vi "OnFontOrLocaleChange.vi"(0 "XRef":T10, 1 "State In":T1 {"BlockNodeState"."Draw Style" items=["FunctionBlock", "ExpressVI", "Variable", "Elemental I/O", "32x32 Icon", "FunctionBlockCompact"]; "BlockNodeState"."Terminal Data"."Terminal Flags" format="%.0b"}) -> (14 "Reply":T8, 15 "State Out":T1 {"BlockNodeState"."Draw Style" items=["FunctionBlock", "ExpressVI", "Variable", "Elemental I/O", "32x32 Icon", "FunctionBlockCompact"]; "BlockNodeState"."Terminal Data"."Terminal Flags" format="%.0b"})   [LabVIEW 2017, in "ExpressFormulaBlockNode.xnode"]
uses:
  <vilib>/express/express arith-compare/Formula/XNode/ExpressFormulaBlockNode.xnode
  <vilib>/XNodeSupport/XNodeXNodeRef.ctl
  <vilib>/express/express arith-compare/Formula/XNode/State.ctl
  <vilib>/BlockNodeSupport/BlockNodeState.ctl
  <vilib>/BlockNodeSupport/TerminalData.ctl
  <vilib>/picture/picture.llb/imagedata.ctl
  <vilib>/express/express shared/XNodes/controls/ExpressState.ctl
  <vilib>/express/express shared/XNodes/controls/ExpressTerminalInfo.ctl
  <vilib>/XNodeSupport/XNodeType.ctl
  <vilib>/XNodeSupport/XNodeStringArray.ctl
  <vilib>/XNodeSupport/XNodeString.ctl
  <vilib>/XNodeSupport/NI_XNodeSupport.lvlib
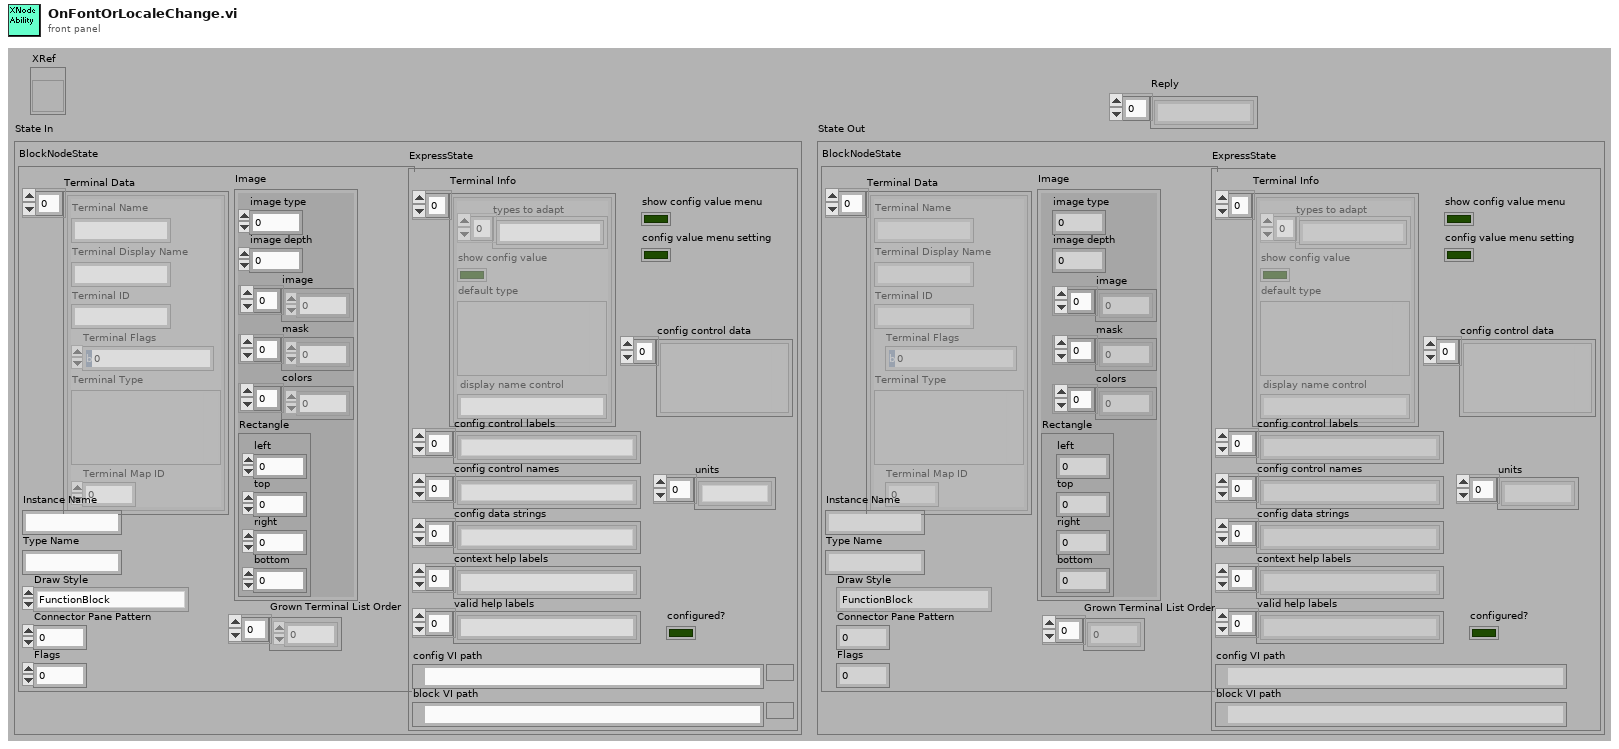
[diagram p1: front panel]
types:
  T1 = typedef "ExpressFormulaBlockNode.xnode/State.ctl" = cluster{"BlockNodeState":T2, "ExpressState":T5}
  T2 = typedef "BlockNodeState.ctl" = cluster{"Terminal Data":T3[], "Instance Name":string, "Type Name":string, "Draw Style":i32, "Connector Pane Pattern":i32, "Flags":i32, "Grown Terminal List Order":i32[], "Image":T4}
  T3 = typedef "TerminalData.ctl" = cluster{"Terminal Name":string, "Terminal Display Name":string, "Terminal ID":string, "Terminal Flags":i32, "Terminal Type":variant, "Terminal Map ID":i32}
  T4 = typedef "imagedata.ctl" = cluster{"image type":i32, "image depth":i32, "image":u8[], "mask":u8[], "colors":u32[], "Rectangle":cluster{"left":i16, "top":i16, "right":i16, "bottom":i16}}
  T5 = typedef "ExpressState.ctl" = cluster{"Terminal Info":T6, "config control names":string[], "config data strings":string[], "config control data":variant[], "units":string[], "configured?":bool, "config VI path":path, "block VI path":path, "config control labels":string[], "show config value menu":bool, "config value menu setting":bool, "context help labels":string[], "valid help labels":string[]}
  T6 = typedef "ExpressTerminalInfo.ctl" = cluster{"types to adapt":string[], "show config value":bool, "default type":T7, "display name control":string}[]
  T7 = typedef "NI_XNodeSupport.lvlib/XNodeType.ctl" = variant
  T8 = typedef "NI_XNodeSupport.lvlib/XNodeStringArray.ctl" = T9[]
  T9 = typedef "NI_XNodeSupport.lvlib/XNodeString.ctl" = string
  T10 = typedef "NI_XNodeSupport.lvlib/XNodeXNodeRef.ctl" = refnum<vi>
  T11 = typedef "ExpressBlockNodeState.ctl" = cluster{"BlockNodeState":T2, "ExpressState":T5}
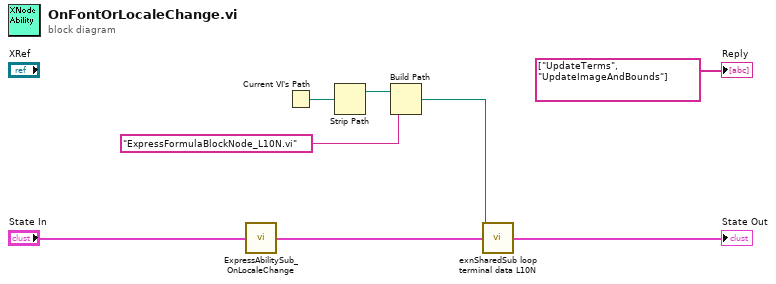
[diagram p0: block diagram]
diagram:
  n1 = call <vilib>:"ExpressAbilitySub_OnLocaleChange.vi"("State In"="State In") -> ("State Out"=w2:T11)  [unwired: 14 in]
  n2 = Current VI's Path() -> (path=w6:path)
  n3 = Strip Path(path=w6) -> (stripped path=w5:path)  [unwired: 1 out]
  n4 = Build Path(base path=w5, name or relative path="ExpressFormulaBlockNode_L10N.vi") -> (appended path=w7:path)
  n5 = call <vilib>:"exnSharedSub loop terminal data L10N.vi"("path to L10N subVI"=w7, "ExpressBlockNodeState In"=w2) -> ("ExpressBlockNodeState Out"=→"State Out":T11)  [unwired: 13 in]
  "Reply" <- T8 ["UpdateTerms", "UpdateImageAndBounds"] ("Reply")
